vi "DSF.Engine.Framework.Initialize.vi"(8 "error in (no error)":errorcluster, 11 "Framework type":refnum<class "DSF.Engine.Framework.lvclass">) -> (0 "error out":errorcluster, 3 "Framework out":refnum<class "DSF.Engine.Framework.lvclass">)   [LabVIEW 2017, in "DSF.Engine.lvlib" / "DSF.Engine.Framework.lvclass"]
uses:
  DSF.Engine.Framework.lvclass
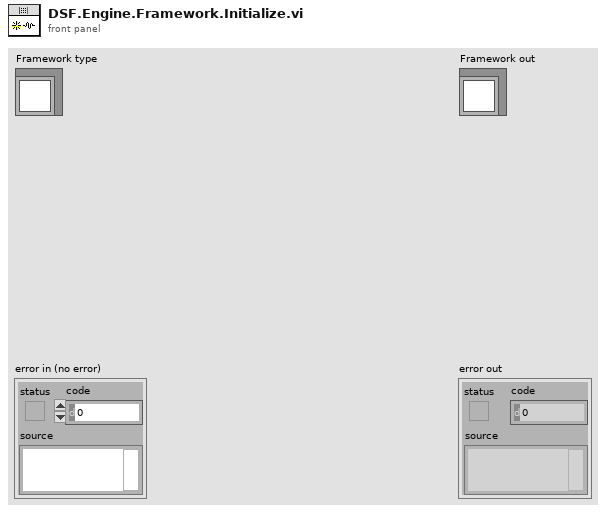
[diagram p1: front panel]
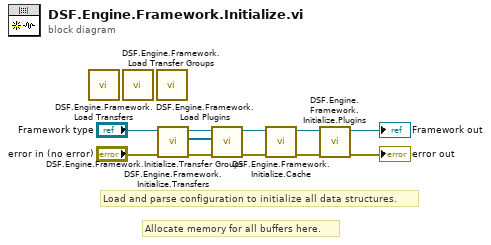
[diagram p0: block diagram]
diagram:
  # "Allocate memory for all buffers here."
  # "Load and parse configuration to initialize all data structures."
  n1 = call "DSF.Engine.Framework.Load Transfers.vi"() -> ()  [unwired: 9 in, 3 out]
  n2 = call "DSF.Engine.Framework.Load Transfer Groups.vi"() -> ()  [unwired: 9 in, 3 out]
  n3 = call "DSF.Engine.Framework.Load Plugins.vi"() -> ()  [unwired: 9 in, 3 out]
  n4 = call "DSF.Engine.Framework.Initialize.Transfers.vi"("error in (no error)"="error in (no error)", "Framework in"="Framework type") -> ("error out"=w8:errorcluster, "All Transfers"=w7:refnum<class "DSF.Engine.Transfer.lvclass">[], "Framework out"=w9:refnum<class "DSF.Engine.Framework.lvclass">)  [unwired: 7 in]
  n5 = call "DSF.Engine.Framework.Initialize.Transfer Groups.vi"("error in (no error)"=w8, "All Transfers"=w7, "Framework in"=w9) -> ("error out"=w3:errorcluster, "Framework out"=w4:refnum<class "DSF.Engine.Framework.lvclass">)  [unwired: 6 in, 1 out]
  n6 = call "DSF.Engine.Framework.Initialize.Cache.vi"("error in (no error)"=w3, "Framework in"=w4) -> ("error out"=w1:errorcluster, "Framework out"=w2:refnum<class "DSF.Engine.Framework.lvclass">)  [unwired: 8 in]
  n7 = call "DSF.Engine.Framework.Initialize.Plugins.vi"("error in (no error)"=w1, "Framework in"=w2) -> ("error out"=→"error out":errorcluster, "Framework out"=→"Framework out":refnum<class "DSF.Engine.Framework.lvclass">)  [unwired: 8 in]
